vi "Parse Bits.vi"(8 "error in (no error)":errorcluster, 11 "Packet in":refnum<class "Packet.lvclass">) -> (0 "error out":errorcluster, 3 "Packet out":refnum<class "Packet.lvclass">)   [LabVIEW 2020, in "Packet.lvclass"]
uses:
  Packet.lvclass
  Type.ctl
  Packet.lvclass/Packet.ctl
  Operator/Operator.lvclass
  C:/dev/IlluminatedG/AdventOfCode/2021/source/Day 16/Part 1/Packet/Packet.lvclass
  Literal/Literal.lvclass
  C:/dev/IlluminatedG/AdventOfCode/2021/source/Day 16/Part 1/Operator/Operator.lvclass
  C:/dev/IlluminatedG/AdventOfCode/2021/source/Day 16/Part 1/Literal/Literal.lvclass
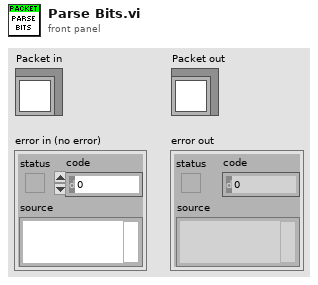
[diagram p1: front panel]
types:
  T1 = typedef "Type.ctl" = enum8{"Unknown", "NA 1", "NA 2", "NA 3", "Literal", "NA 5", "NA 6"}
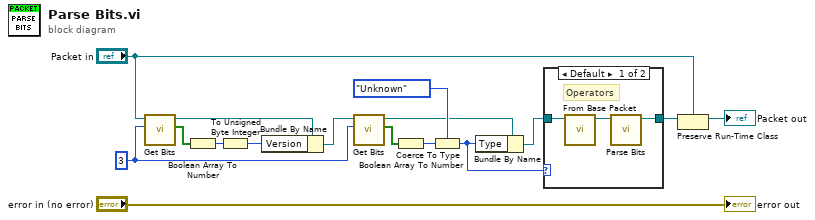
[diagram p0: block diagram]
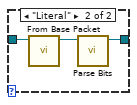
[diagram p2: hidden frame]
diagram:
  w11 = 3 ("Count (1)")
  n1 = call "Get Bits.vi"("Count (1)"=w11, "Packet in"="Packet in") -> ("Bits"=w16:bool[], "Packet out"=w13:refnum<class "Packet.lvclass">)  [unwired: 7 in, 1 out]
  n2 = Boolean Array To Number(Boolean array=w16) -> (number=w15:u32)
  n3 = To Unsigned Byte Integer(number=w15) -> (unsigned 8bit integer=w14:u8)
  n4 = Bundle By Name(cluster=w13, "Version"=w14) -> (w12:refnum<class "Packet.lvclass">)
  n5 = call "Get Bits.vi"("Count (1)"=w11, "Packet in"=w12) -> ("Bits"=w10:bool[], "Packet out"=w7:refnum<class "Packet.lvclass">)  [unwired: 7 in, 1 out]
  n6 = Boolean Array To Number(Boolean array=w10) -> (number=w9:u32)
  n7 = Coerce To Type(0:w9, 1:Type."Unknown" ("Type")) -> (2:w5:T1)
  n8 = Bundle By Name(cluster=w7, "Type"=w5) -> (w6:refnum<class "Packet.lvclass">)
  n9 = case shown="Default" w5 {
    tunnel: w6 -> [w19 w22]
    tunnel: [w17 w20] -> w3
    frame Default {
      # "Operators"
      n10 = call "From Base Packet.vi"("Base Packet"=w19) -> ("Operator out"=w18:refnum<class "Operator.lvclass">)  [unwired: 9 in, 1 out]
      n11 = call-dynamic "Parse Bits.vi"("Operator in"=w18) -> ("Operator out"=w17:refnum<class "Operator.lvclass">)  [unwired: 9 in, 1 out]
    }
    frame "Literal" {
      n12 = call "From Base Packet.vi"("Base Packet"=w22) -> ("Literal out"=w21:refnum<class "Literal.lvclass">)  [unwired: 9 in, 1 out]
      n13 = call-dynamic "Parse Bits.vi"("Literal in"=w21) -> ("Literal out"=w20:refnum<class "Literal.lvclass">)  [unwired: 9 in, 1 out]
    }
  }
  n14 = Preserve Run-Time Class(object in=w3, 2:"Packet in") -> (object out=→"Packet out":refnum<class "Packet.lvclass">)  [unwired: 1 in, 1 out]
  "error out" <- "error in (no error)"
